vi "CheckAcPwrParamLoopCondition.vi"(8 "ErrorArray":errorcluster[](array[cluster]), 11 "AcPwrLoopingCtrl":T1) -> (0 "ErrorArrayOut":errorcluster[](array[cluster]), 3 "AcPwrLoopingCtrl out":T1)   [LabVIEW 2018, in "Test.lvclass"]
uses:
  Test.lvclass
  AcPwr/AcPwrPlugins/AcPwrBaseClass/TypeDefs/AcPwrSSMLoopingCtrl.ctl
  AcPwr/AcPwrPlugins/AcPwrPlugins.lvlib
  AcPwr/AcPwrPlugins/AcPwrBaseClass/AcPwrBase.lvclass
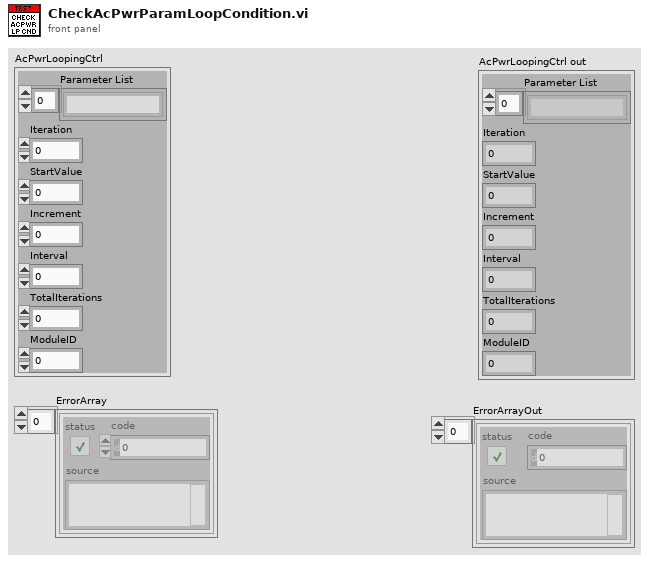
[diagram p1: front panel]
types:
  T1 = typedef "AcPwrPlugins.lvlib/AcPwrBase.lvclass/AcPwrSSMLoopingCtrl.ctl" = cluster{"Parameter List":string[], "Iteration":u32, "StartValue":dbl, "Increment":dbl, "Interval":dbl, "TotalIterations":u32, "ModuleID":i32}
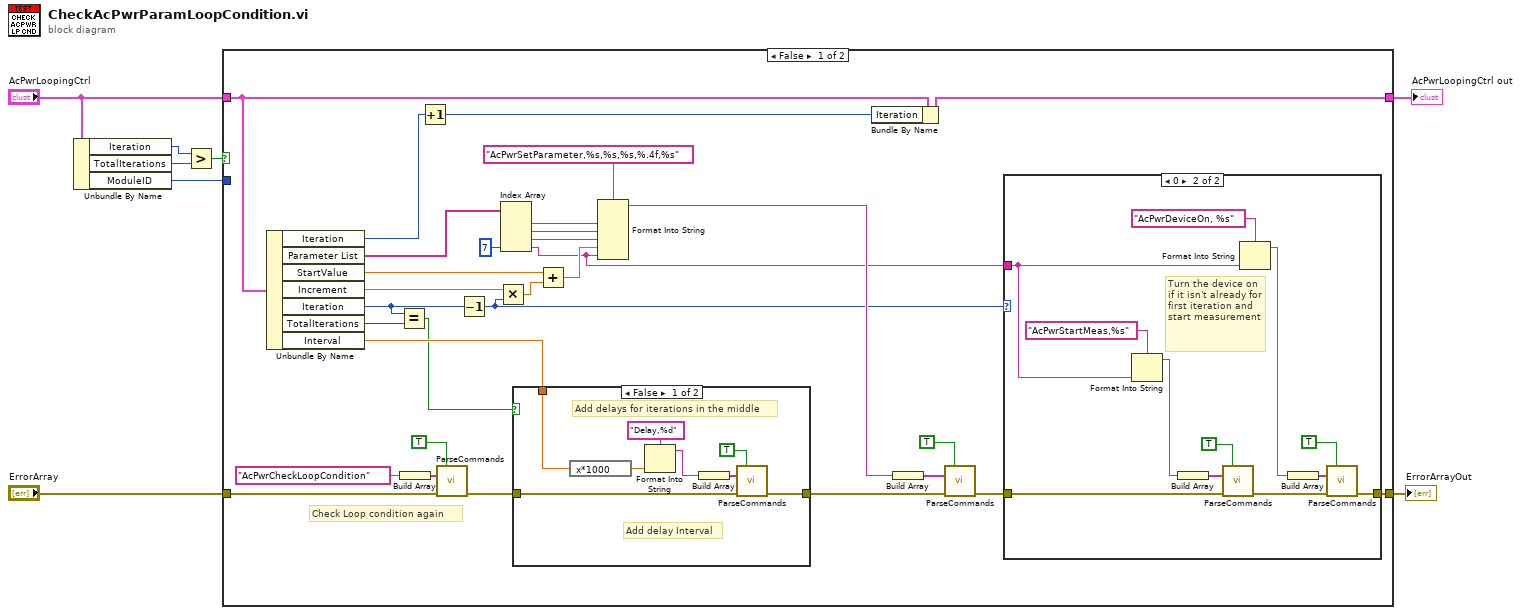
[diagram p0: block diagram]
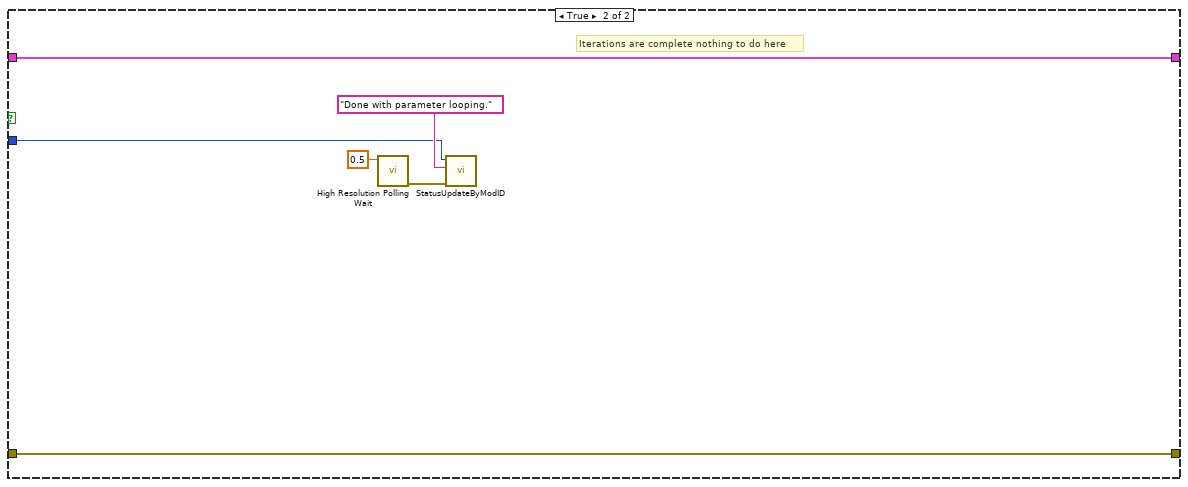
[diagram p4: hidden frame]
diagram:
  n1 = Unbundle By Name("AcPwrLoopingCtrl") -> ("Iteration"=w4:u32, "TotalIterations"=w3:u32, "ModuleID"=w1:i32)
  n2 = Greater?(x=w4, y=w3) -> (0:w2:bool)
  n3 = case shown="False" w2 {
    tunnel: "ErrorArray" -> [w13 w66]
    tunnel: [w21 w67] -> w7
    tunnel: [w18 w66] -> w6
    tunnel: "AcPwrLoopingCtrl" -> [w15 w67]
    tunnel: w1 -> [_ w62]
    frame False {
      # "Check Loop condition again"
      n4 = Unbundle By Name(w15) -> ("Iteration"=w23:u32, "Parameter List"=w25:string[], "StartValue"=w32:dbl, "Increment"=w31:dbl, "Iteration"=w9:u32, "TotalIterations"=w36:u32, "Interval"=w37:dbl)
      n5 = Equal?(x=w9, y=w36) -> (x = y?=w20:bool)
      n6 = Build Array("AcPwrCheckLoopCondition" ("String")) -> (w10:string[])
      n7 = Increment(x=w23) -> (x+1=w22:u32)
      n8 = call "ParseCommands.vi"("Priority? (f)"=TRUE, "Script In"=w10, "ErrorArrayIn"=w13) -> ("ErrorArrayOut"=w12:errorcluster[])  [unwired: 11 in, 1 out]
      n9 = Decrement(x=w9) -> (x-1=w17:u32)
      n10 = Multiply(x=w31, y=w17) -> (x*y=w30:dbl)
      n11 = Index Array(array=w25, index #4=7 ("index")) -> (element #1=w27:string, element #2=w28:string, element #3=w29:string, element #4=w16:string)  [unwired: 3 in]
      n12 = case shown="False" w20 {
        tunnel: w12 -> [w47 w48]
        tunnel: w37 -> [w46 _]
        tunnel: [w45 w48] -> w35
        frame False {
          # "Add delays for iterations in the middle"
          # "Add delay Interval"
          n13 = expression code="x*1000"(w46) -> (w43:dbl)
          n14 = Format Into String(format string="Delay,%d", w43) -> (resulting string=w42:string)  [unwired: 2 in, 1 out]
          n15 = Build Array(w42) -> (w40:string[])
          n16 = call "ParseCommands.vi"("Priority? (f)"=TRUE, "Script In"=w40, "ErrorArrayIn"=w47) -> ("ErrorArrayOut"=w45:errorcluster[])  [unwired: 11 in, 1 out]
        }
        frame True {
        }
      }
      n17 = Add(x=w32, y=w30) -> (x+y=w33:dbl)
      n18 = Format Into String(format string="AcPwrSetParameter,%s,%s,%s,%.4f,%s", w27, w28, w29, w33, w16) -> (resulting string=w38:string)  [unwired: 2 in, 1 out]
      n19 = Bundle By Name(cluster=w15, "Iteration"=w22) -> (w21:T1)
      n20 = Build Array(w38) -> (w39:string[])
      n21 = call "ParseCommands.vi"("Priority? (f)"=TRUE, "Script In"=w39, "ErrorArrayIn"=w35) -> ("ErrorArrayOut"=w19:errorcluster[])  [unwired: 11 in, 1 out]
      n22 = case shown="0" w17 {
        tunnel: w19 -> [w49 w56]
        tunnel: [w49 w60] -> w18
        tunnel: w16 -> [_ w50]
        frame Default {
        }
        frame 0 {
          # "Turn the device on if it isn't already for first iteration and start measurement"
          n23 = Format Into String(format string="AcPwrStartMeas,%s", w50) -> (resulting string=w52:string)  [unwired: 2 in, 1 out]
          n24 = Build Array(w52) -> (w51:string[])
          n25 = call "ParseCommands.vi"("Priority? (f)"=TRUE, "Script In"=w51, "ErrorArrayIn"=w56) -> ("ErrorArrayOut"=w55:errorcluster[])  [unwired: 11 in, 1 out]
          n26 = Format Into String(format string="AcPwrDeviceOn, %s", w50) -> (resulting string=w58:string)  [unwired: 2 in, 1 out]
          n27 = Build Array(w58) -> (w57:string[])
          n28 = call "ParseCommands.vi"("Priority? (f)"=TRUE, "Script In"=w57, "ErrorArrayIn"=w55) -> ("ErrorArrayOut"=w60:errorcluster[])  [unwired: 11 in, 1 out]
        }
      }
    }
    frame True {
      # "Iterations are complete nothing to do here"
      n29 = call <vilib>:"High Resolution Polling Wait.vi"("seconds to wait"=0.5) -> ("error out"=w64:errorcluster)  [unwired: 10 in]
      n30 = call "StatusUpdateByModID.vi"("error in (no error)"=w64, "Status"="Done with parameter looping.", "Accessors:Module ID"=w62) -> ()  [unwired: 8 in, 1 out]
    }
  }
  "ErrorArrayOut" <- w6
  "AcPwrLoopingCtrl out" <- w7
